vi "OAT Continuous Waterfall Plot.vi"(5 "reset? (True)":bool=TRUE, 6 "plot settings":T2={"plot color"=65280, "max Z range"=11, "X shift (rel to total X)"=0.1, "number of spectra"=40} {"X shift (rel to total X)" format="%.2f"; "max Z range" items=["10^-7", "10^-6", "10^-5", "0.0001", "0.001", "0.01", "0.1", "1", "10", "100", "1000", "auto z range"]}, 7 "waterfall plot ref":refnum<vi>, 8 "error in (no error)":errorcluster, 9 "unit labels":T1, 10 "scales":T3 {"Y scale"."multiplier" format="%.2f"; "Y scale"."offset" format="%.2f"; "X scale"."multiplier" format="%.2f"; "X scale"."offset" format="%.2f"}, 11 "spectral map":dbl[][](array[numeric]) format="%.2f") -> (0 "error out":errorcluster, 3 "waterfall plot":cluster{"X0":dbl, "dX":dbl, "Y":dbl[]}[](array[cluster]) {"Y" format="%.2f"; "dX" format="%.2f"; "X0" format="%.2f"})   [LabVIEW 2017]
doc: "Receives <B>spectral map</B> from the OAT Online Spectral Map with Resample VI and continuously displays the data in a waterfall plot."
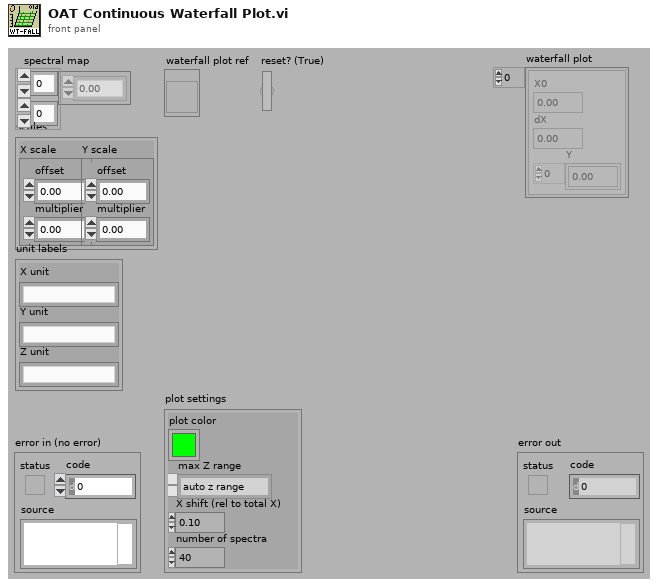
[diagram p1: front panel]
types:
  T1 = cluster{"X unit":string, "Y unit":string, "Z unit":string}
  T2 = cluster{"plot color":u32, "max Z range":u16, "X shift (rel to total X)":dbl, "number of spectra":i32}
  T3 = cluster{"X scale":cluster{"offset":dbl, "multiplier":dbl}, "Y scale":cluster{"offset":dbl, "multiplier":dbl}}
  T4 = cluster{"plot color":u32, "plot color":u32, "X shift (rel to total X)":dbl, "max Z range":u16, "number of spectra":i32}
  T5 = cluster{"num of displayed spectra":i32, "num of new spectra":i32}
  T6 = cluster{"plot color":u32, "grid color":u32, "X shift (rel to total X)":dbl, "max Z range":u16, "number of spectra":i32}
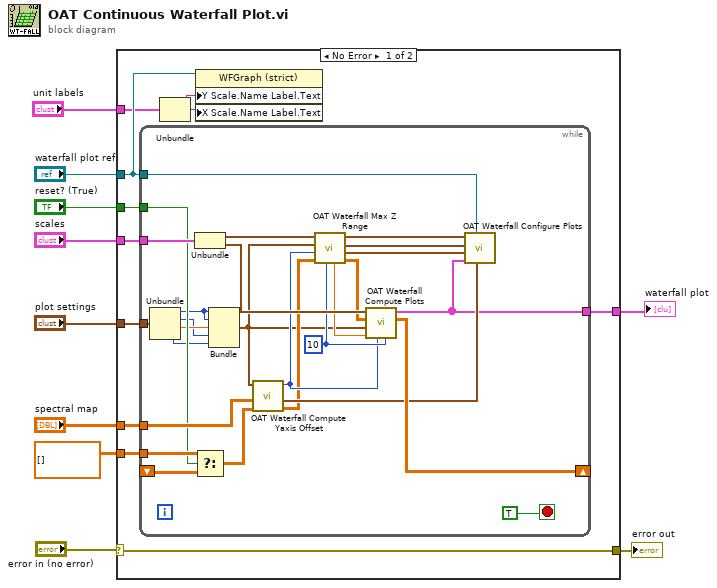
[diagram p0: block diagram]
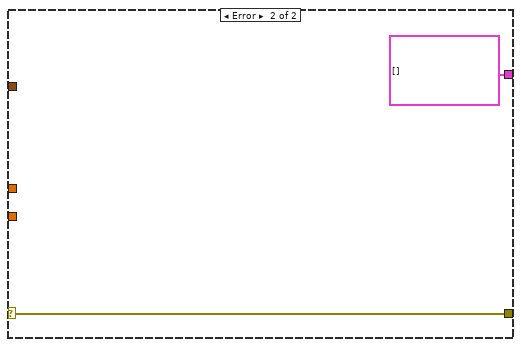
[diagram p2: hidden frame]
diagram:
  n1 = case shown="No Error" "error in (no error)" {
    selector: "error in (no error)" -> [w12 w50]
    tunnel: "scales" -> [w21 _]
    tunnel: "spectral map" -> [w20 _]
    tunnel: "reset? (True)" -> [w19 _]
    tunnel: dbl[][] [] -> [w18 _]
    tunnel: "plot settings" -> [w17 _]
    tunnel: "waterfall plot ref" -> [w14 _]
    tunnel: "unit labels" -> [w13 _]
    tunnel: [w12 w50] -> w2
    tunnel: [w11 cluster{"X0":dbl, "dX":dbl, "Y":dbl[]}[] [] ("waterfall plot")] -> w1
    frame No Error {
      n2 = while {
        shift-right: [w42] -> _
        shift-left: _ -> [w48]
        tunnel: w21 -> [w47]
        tunnel: w20 -> [w40]
        tunnel: w19 -> [w29]
        tunnel: w18 -> [w45]
        tunnel: w17 -> [w27]
        tunnel: w14 -> [w39]
        tunnel: [w28] -> w11
        stop <- TRUE stop-if-true
        w36 = 10 ("zoom factor")
        n3 = Unbundle(w27) -> ("plot color"=w26:u32, "max Z range"=w22:u16, "X shift (rel to total X)"=w23:dbl, "number of spectra"=w25:i32)
        n4 = Unbundle(w47) -> ("X scale"=w44:cluster{"offset":dbl, "multiplier":dbl}, "Y scale"=w43:cluster{"offset":dbl, "multiplier":dbl})
        n5 = Select(t=w45, s=w29, f=w48) -> (s? t:f=w41:dbl[][])
        n6 = Bundle("plot color"=w26, "plot color"=w26, "X shift (rel to total X)"=w23, "max Z range"=w22, "number of spectra"=w25) -> (w24:T4)  [unwired: 1 in]
        n7 = call <vilib>:"OAT Waterfall Compute Yaxis Offset.vi"("spectral map history"=w41, "spectral map new"=w40, "plot settings"=w24) -> ("spectral map for display"=w32:dbl[][], "spectra info"=w37:T5, "Y axis offset"=w34:i32)  [unwired: 6 in]
        n8 = call <vilib>:"OAT Waterfall Max Z Range.vi"("zoom factor"=w36, "spectral map in"=w32, "Y axis offset"=w34, "plot settings"=w24, "scale in"=w44) -> ("spectral map out"=w31:dbl[][], "Y range"=w35:cluster{"min":dbl, "max":dbl}, "plot settings"=w30:T6, "scale out"=w38:cluster{"offset":dbl, "multiplier":dbl}, "max Z range"=w33:dbl)  [unwired: 2 in]
        n9 = call <vilib>:"OAT Waterfall Compute Plots.vi"("zoom factor"=w36, "Y axis offset"=w34, "max Z range"=w33, "plot settings"=w24, "spectral map in"=w31, "X scale"=w43) -> ("spectral map out"=w42:dbl[][], "waterfall plot"=w28:cluster{"X0":dbl, "dX":dbl, "Y":dbl[]}[])  [unwired: 2 in, 2 out]
        n10 = call <vilib>:"OAT Waterfall Configure Plots.vi"("spectra info"=w37, "reference"=w39, "waterfall plot"=w28, "Y range"=w35, "plot settings"=w30, "Y scale"=w38) -> ()  [unwired: 5 in, 1 out]
      }
      n11 = Unbundle(w13) -> ("X unit"=w16:string, "Y unit"=w15:string)  [unwired: 1 out]
      n12 = property on="Property Node" class="WFGraph (strict)"(reference=w14, "Y Scale.Name Label.Text"=w16, "X Scale.Name Label.Text"=w15) -> ()  [unwired: 1 in, 2 out]
    }
    frame Error {
    }
  }
  "error out" <- w2
  "waterfall plot" <- w1
